vi "Reporter_Create.vi"(0 "reference in":refnum<class "Reporter.lvclass">, 5 "error in (no error)":errorcluster, 6 "LCR":refnum<class "BKP-891 LCR Meter.lvclass">, 8 "PSU":refnum<class "BKP-911x Power Supply.lvclass">, 10 "NI-DAQmx":refnum<class "NI-DAQmx.lvclass">) -> (14 "reference out":refnum<class "Reporter.lvclass">, 19 "error out":errorcluster)   [LabVIEW 2018, in "Reporter.lvclass"]
uses:
  Reporter.lvclass
  BKP-891 LCR Meter_class/BKP-891 LCR Meter.lvclass
  BKP-911x Power Supply_class/BKP-911x Power Supply.lvclass
  NI-DAQmx_class/NI-DAQmx.lvclass
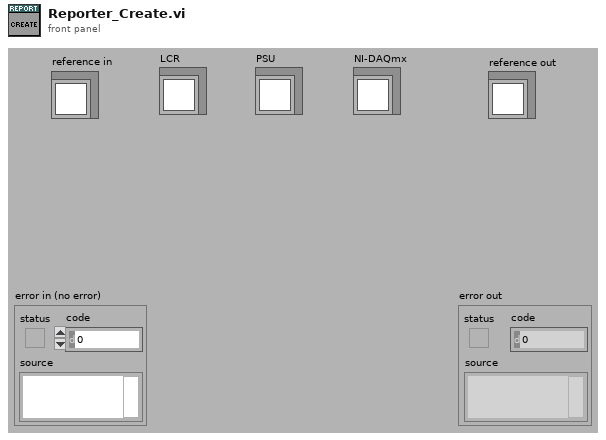
[diagram p1: front panel]
types:
  T1 = typedef "VI-TechBaseTemplate_Simple_6x8x6.lvclass/ObjectAttributes.ctl" = cluster{"Attribute1":dbl}
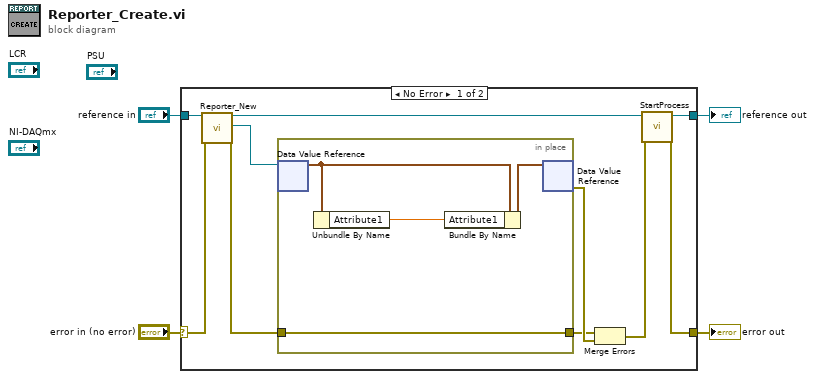
[diagram p0: block diagram]
diagram:
  n1 = case shown="No Error" "error in (no error)" {
    selector: "error in (no error)" -> [w13 w20]
    tunnel: [w5 w20] -> w3
    tunnel: "reference in" -> [w14 w19]
    tunnel: [w7 w19] -> w1
    frame No Error {
      n2 = call "Reporter_New.vi"("reference in"=w14, "error in (no error)"=w13) -> ("reference out"=w8:refnum<class "Reporter.lvclass">, "DVRRefOut"=w11:refnum<data-value>, "error out"=w10:errorcluster)  [unwired: 14 in, 1 out]
      n3 = in-place {
        in-place-border: w10 -> [w15]
        in-place-border: [w15] -> w9
        n4 = in-place-dvr #1(w11) -> (w17:T1)  [unwired: 1 out]
        n5 = Unbundle By Name(w17) -> ("Attribute1"=w16:dbl)
        n6 = Bundle By Name(cluster=w17, "Attribute1"=w16) -> (w18:T1)
        n7 = in-place-dvr #1(w18) -> (w12:errorcluster)  [unwired: 1 out]
      }
      n8 = Merge Errors(w9, w12) -> (w6:errorcluster)
      n9 = call "StartProcess.vi"("reference in"=w8, "error in (no error)"=w6) -> ("reference out"=w7:refnum<class "Reporter.lvclass">, "error out"=w5:errorcluster)  [unwired: 14 in, 2 out]
    }
    frame Error {
      # "VI-TechBaseTemplate_Simple_6x8x6"
    }
  }
  "error out" <- w3
  "reference out" <- w1
